vi "Initialize.vi"(6 "Parameters":T1[](array[typedef]) {"Base Word" format="%04d"}, 8 "error in (no error)":errorcluster, 10 "Filter Configuration":T3={"Filter Type"=enum."Transmit", "Terminal Address (0-30)"=enum."0", "SubAddress (1-30)"=enum."1", "Mode Code"=FALSE, "Broadcast"=FALSE, "RT-RT"=FALSE, "Bus A"=FALSE}, 11 "ID":string) -> (0 "error out":errorcluster, 3 "Filter out":refnum<class "Filter.lvclass">)   [LabVIEW 2020, in "BCI-1553 API.lvlib" / "Filter.lvclass"]
doc: "Creates a Filter object that can be added to a Bus Monitor."
uses:
  Filter.lvclass
  TypeDefs/Filter Configuration.ctl
  Frames & Messages/TypeDefs/Command Type.ctl
  Frames & Messages/TypeDefs/Command Terminal Address.ctl
  Frames & Messages/TypeDefs/Command SubAddress.ctl
  Frames & Messages/TypeDefs/Simplified Parameter Data Table.ctl
  Frames & Messages/TypeDefs/Scaling Information.ctl
  Frames & Messages/TypeDefs/Parameter Table Data.ctl
  Filter.lvclass/Filter.ctl
  BCI-1553 API.lvlib
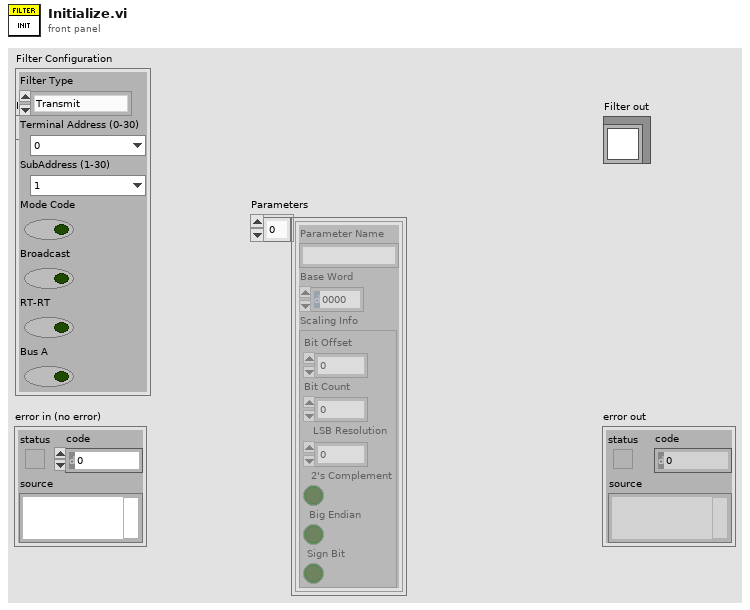
[diagram p1: front panel]
types:
  T1 = typedef "BCI-1553 API.lvlib/Simplified Parameter Data Table.ctl" = cluster{"Parameter Name":string, "Base Word":u16, "Scaling Info":T2}
  T2 = typedef "BCI-1553 API.lvlib/Scaling Information.ctl" = cluster{"Bit Offset":i32, "Bit Count":i32, "LSB Resolution":dbl, "2's Complement":bool, "Big Endian":bool, "Sign Bit":bool}
  T3 = typedef "BCI-1553 API.lvlib/Filter Configuration.ctl" = cluster{"Filter Type":T4, "Terminal Address (0-30)":T5, "SubAddress (1-30)":T6, "Mode Code":bool, "Broadcast":bool, "RT-RT":bool, "Bus A":bool}
  T4 = typedef "BCI-1553 API.lvlib/Command Type.ctl" = enum16{"Transmit", "Receive"}
  T5 = typedef "BCI-1553 API.lvlib/Command Terminal Address.ctl" = enum16{"0", "1", "2", "3", "4", "5", "6", "7", "8", "9", "10", "11", "12", "13", "14", "15", "16", "17", "18", "19", "20", "21", "22", "23", "24", "25", "26", "27", "28", "29", "30", "Broadcast"}
  T6 = typedef "BCI-1553 API.lvlib/Command SubAddress.ctl" = enum16{"Mode Code", "1", "2", "3", "4", "5", "6", "7", "8", "9", "10", "11", "12", "13", "14", "15", "16", "17", "18", "19", "20", "21", "22", "23", "24", "25", "26", "27", "28", "29", "30"}
  T7 = typedef "BCI-1553 API.lvlib/Parameter Table Data.ctl" = cluster{"Parameter Name":string, "Base Word":u16, "Address":u16, "Value":u64, "Mask":u16[], "Scaling Info":T2}
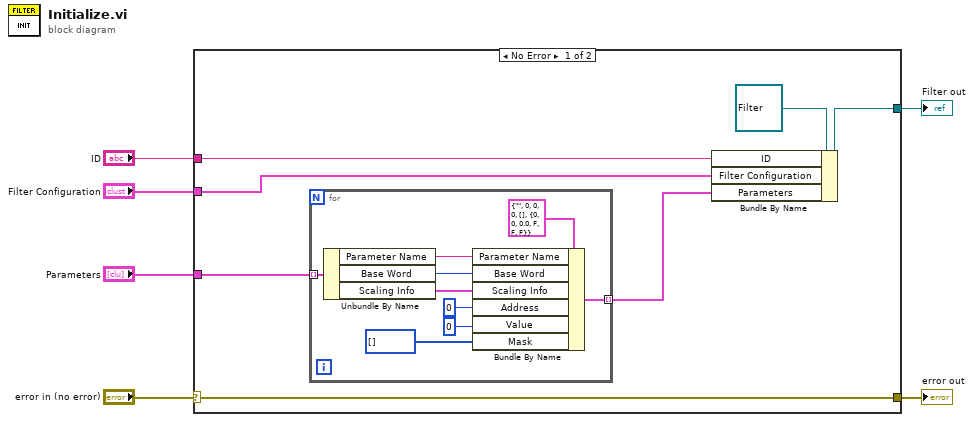
[diagram p0: block diagram]
diagram:
  n1 = case shown="No Error" "error in (no error)" {
    selector: "error in (no error)" -> [w13 w23]
    tunnel: [w13 w23] -> w5
    tunnel: [w11 _] -> w4
    tunnel: "ID" -> [w10 _]
    tunnel: "Filter Configuration" -> [w9 _]
    tunnel: "Parameters" -> [w8 _]
    frame No Error {
      n2 = for {
        tunnel: w8 -> [w20] mode=indexing
        tunnel: [w21] -> w7 mode=indexing
        n3 = Unbundle By Name(w20) -> ("Parameter Name"=w19:string, "Base Word"=w18:u16, "Scaling Info"=w14:T2)
        n4 = Bundle By Name(cluster=T7 {"Parameter Name"="", "Base Word"=0, "Address"=0, "Value"=0, "Mask"=[], "Scaling Info"={"Bit Offset"=0, "Bit Count"=0, "LSB Resolution"=0.0, "2's Complement"=FALSE, "Big Endian"=FALSE, "Sign Bit"=FALSE}} ("Parameter Table Data"), "Parameter Name"=w19, "Base Word"=w18, "Scaling Info"=w14, "Address"=u16 0, "Value"=u64 0, "Mask"=u16[] []) -> (w21:T7)
      }
      n5 = Bundle By Name(cluster=refnum<class "Filter.lvclass"> refnum ("Filter out"), "ID"=w10, "Filter Configuration"=w9, "Parameters"=w7) -> (w11:refnum<class "Filter.lvclass">)
    }
    frame Error {
    }
  }
  "error out" <- w5
  "Filter out" <- w4
